vi "testVI.vi"() -> ()   [LabVIEW 2017]
panel:
  in  "String":string
  out "Slide 2":u8(slide) scale=0.0..100.0
  in  "Slide":i32(slide) scale=0.0..10.0
  out "Numeric 2":dbl
  in  "Numeric":i32 format="%.0x"
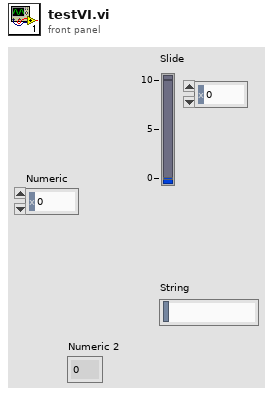
[diagram p1: front panel]
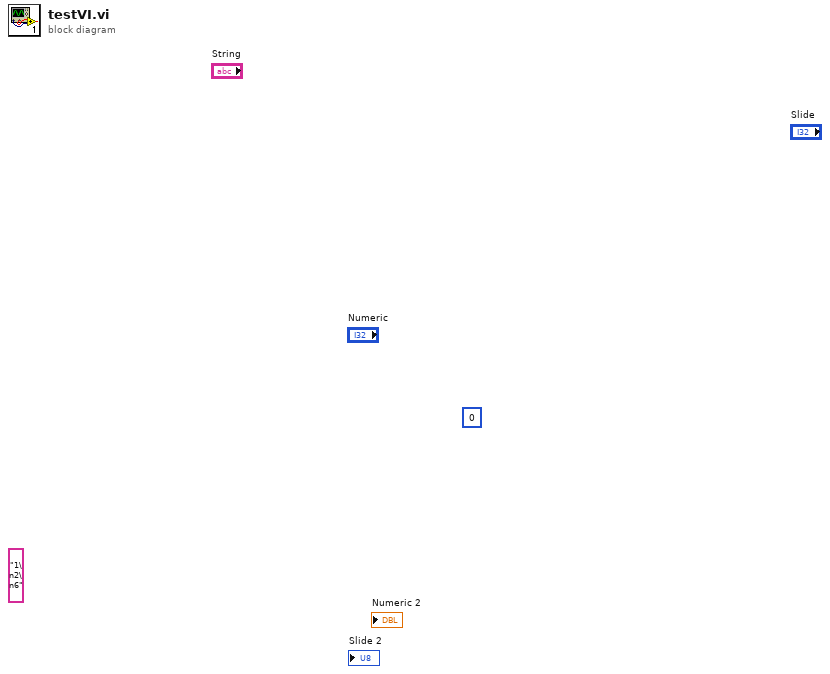
[diagram p0: block diagram]
diagram:
  (unwired) "1\n2\n6"
  (unwired) 0 ("Signed 32-bit integer")
